vi "Sirene.vi"() -> ()   [LabVIEW 2019]
uses:
  <vilib>/sound2/lvsound2.llb/Sound File Info (path).vi
panel:
  out "appended path":path
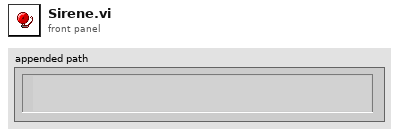
[diagram p1: front panel]
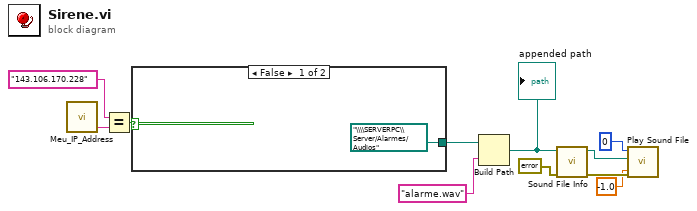
[diagram p0: block diagram]
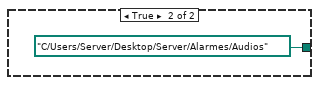
[diagram p2: hidden frame]
diagram:
  n1 = call "Meu_IP_Address.vi"() -> ("Meu IP"=w4:string)  [unwired: 4 in, 1 out]
  n2 = Equal?(x="143.106.170.228", y=w4) -> (x = y?=w2:bool)
  n3 = case shown="False" w2 {
    tunnel: [path "\\\\SERVERPC\\Server/Alarmes/Audios" ("base path") path "C:/Users/Server/Desktop/Server/Alarmes/Audios" ("base path")] -> w1
    frame False {
    }
    frame True {
    }
  }
  n4 = Build Path(base path=w1, name or relative path="alarme.wav") -> (appended path=w10:path)
  "appended path" <- w10
  n5 = call-poly <vilib>:"Sound File Info.vi"("error in (no error)"=errorcluster {"status"=FALSE, "code"=0, "source"=""}, "path"=w10) -> ("error out"=w9:errorcluster, "path out"=w5:path)  [unwired: 6 in, 2 out]
  n6 = call <vilib>:"Play Sound File.vi"("timeout (sec)"=-1.0, "error in (no error)"=w9, "path"=w5, "device ID"=u32 0) -> ()  [unwired: 6 in, 2 out]
